vi "Lab Panel V4.83.vi"() -> ()   [LabVIEW 2013] (continued)
                        n911 = Number To Decimal String(number=w1505) -> (decimal integer string=w1518:string)  [unwired: 1 in]
                        n912 = Number To Decimal String(number=w1504) -> (decimal integer string=w1517:string)  [unwired: 1 in]
                        n913 = Number To Decimal String(number=w1503) -> (decimal integer string=w1516:string)  [unwired: 1 in]
                        n914 = Build Array(w1507, w1506, w1518, w1517, w1516) -> (w1515:string[])
                        n915 = TDMS Set Properties(5:w1515, 7:w1509, 11:w1519) -> ()  [unwired: 3 in, 4 out]
                      }
                      frame #3 {
                        w1521 = 0.0
                        n916 = local read "DISP LAB05-2"() -> (w1523:T4)
                        n917 = Bundle(cluster=w1523, "CYCLE"=w1521, "MINS"=w1521, "STATUS"="RUN") -> (w1522:T4)
                        n918 = local write "DISP LAB05-2"(w1522) -> ()
                      }
                      frame #4 {
                        n919 = local read "SIG LAB05-2"() -> (w1526:T2)
                        n920 = local read "TEMP START LAB05-2"() -> (w1528:cluster{"TL":dbl, "TN":dbl})
                        n921 = Unbundle(w1526) -> ("Tmp Live"=w1525:dbl, "Tmp Neut"=w1524:dbl)  [unwired: 3 out]
                        n922 = Bundle(cluster=w1528, "TL"=w1525, "TN"=w1524) -> (w1527:cluster{"TL":dbl, "TN":dbl})
                        n923 = local write "TEMP START LAB05-2"(w1527) -> ()
                      }
                    }
                  }
                }
              }
            }
            n924 = local write "data file error"(w580) -> ()
          }
          frame #4 {
            # "check if test cycles reached for cycle tests, if so then test pass"
            n925 = stacked-sequence {
              tunnel: w1548 -> [_ _ _ _ _ _ _ _ _ _]
              tunnel: w1547 -> [_ _ _ _ _ _ _ _ _ _]
              tunnel: w1546 -> [_ _ _ _ _ _ _ _ _ _]
              tunnel: w1545 -> [_ _ _ _ _ _ _ _ _ _]
              tunnel: w1544 -> [_ _ _ _ _ _ _ _ _ _]
              tunnel: w1543 -> [_ _ _ _ _ _ _ _ _ _]
              tunnel: w1542 -> [_ _ _ _ _ _ _ _ _ _]
              tunnel: w1541 -> [_ _ _ _ _ _ _ _ _ _]
              tunnel: w1540 -> [_ _ _ _ _ _ _ _ _ _]
              tunnel: w1539 -> [_ _ _ _ _ _ _ _ _ _]
              tunnel: w1538 -> [w1554 _ _ _ _ _ _ _ _ _]
              tunnel: w1537 -> [_ w1589 _ _ _ _ _ _ _ _]
              tunnel: w1536 -> [_ _ w1629 _ _ _ _ _ _ _]
              tunnel: w1535 -> [_ _ _ w1669 _ _ _ _ _ _]
              tunnel: w1534 -> [_ _ _ _ w1709 _ _ _ _ _]
              tunnel: w1533 -> [_ _ _ _ _ w1749 _ _ _ _]
              tunnel: w1532 -> [_ _ _ _ _ _ w1789 _ _ _]
              tunnel: w1531 -> [_ _ _ _ _ _ _ w1829 _ _]
              tunnel: w1530 -> [_ _ _ _ _ _ _ _ w1869 _]
              tunnel: w1529 -> [_ _ _ _ _ _ _ _ _ w1909]
              frame #0 {
                # "LAB01-1"
                n926 = Less?(x=w1554, y=2) -> (x < y?=w1552:bool)
                n927 = local read "DISP LAB01-1"() -> (w1555:T4)
                n928 = Unbundle(w1555) -> ("STATUS"=w1549:string)  [unwired: 2 out]
                n929 = Equal?(x=w1549, y="RUN") -> (x = y?=w1551:bool)
                n930 = And(x=w1551, y=w1552) -> (x .and. y?=w1550:bool)
                n931 = case shown="True" w1550 {
                  tunnel: w1555 -> [_ w1560]
                  tunnel: w1554 -> [_ w1564]
                  frame False {
                  }
                  frame True {
                    n932 = local read "SET LAB01-1"() -> (w1566:T5)
                    n933 = local read "TDMS LAB01-1"() -> (w1559:refnum<k34>)
                    n934 = Unbundle(w1566) -> ("CYCLES"=w1557:dbl, "T-RISE mins"=w1563:dbl)  [unwired: 3 out]
                    n935 = case shown="\"CYCLE TEST\"" w1564 {
                      tunnel: w1563 -> [_ _ w1573]
                      tunnel: [w1568 w1570 w1573] -> w1562
                      tunnel: w1557 -> [w1568 w1570 _]
                      tunnel: ["CHART PASS" "CYCLE PASS" "T-RISE PASS"] -> w1561
                      frame "CHART TEST", Default {
                      }
                      frame "CYCLE TEST" {
                      }
                      frame "T-RISE TEST" {
                      }
                    }
                    n936 = Unbundle(w1560) -> ("CYCLE"=w1565:dbl)  [unwired: 2 out]
                    n937 = Increment(x=w1557) -> (x+1=w1558:dbl)
                    n938 = Greater Or Equal?(x=w1565, y=w1558) -> (x >= y?=w1567:bool)
                    n939 = case shown="True" w1567 {
                      tunnel: w1562 -> [w1577 _]
                      tunnel: w1561 -> [w1576 _]
                      tunnel: w1560 -> [w1575 _]
                      tunnel: w1559 -> [w1574 _]
                      frame True {
                        n940 = stacked-sequence {
                          tunnel: w1577 -> [w1581 _]
                          tunnel: w1576 -> [w1579 w1585]
                          tunnel: w1575 -> [_ w1588]
                          tunnel: w1574 -> [w1578 _]
                          frame #0 {
                            n941 = Build Array(w1579) -> (w1582:string[])
                            n942 = Build Array(w1581) -> (w1580:dbl[])
                            n943 = TDMS Write(0:w1578, 5:"TEST PASS", 7:w1582, 9:w1580) -> (15:w1584:errorcluster)  [unwired: 2 in, 3 out]
                            n944 = local write "data file error"(w1584) -> ()
                          }
                          frame #1 {
                            n945 = Bundle(cluster=w1588, "STATUS"=w1585) -> (w1586:T4)  [unwired: 2 in]
                            n946 = local write "RESULT LAB01-1"(TRUE) -> ()
                            n947 = local write "DISP LAB01-1"(w1586) -> ()
                          }
                        }
                      }
                      frame False {
                      }
                    }
                  }
                }
              }
              frame #1 {
                # "LAB01-2"
                n948 = Less?(x=w1589, y=2) -> (x < y?=w1592:bool)
                n949 = local read "DISP LAB01-2"() -> (w1594:T4)
                n950 = Unbundle(w1594) -> ("STATUS"=w1595:string)  [unwired: 2 out]
                n951 = Equal?(x=w1595, y="RUN") -> (x = y?=w1591:bool)
                n952 = And(x=w1591, y=w1592) -> (x .and. y?=w1590:bool)
                n953 = case shown="True" w1590 {
                  tunnel: w1594 -> [_ w1600]
                  tunnel: w1589 -> [_ w1604]
                  frame False {
                  }
                  frame True {
                    n954 = local read "SET LAB01-2"() -> (w1606:T5)
                    n955 = local read "TDMS LAB01-2"() -> (w1599:refnum<k34>)
                    n956 = Unbundle(w1606) -> ("CYCLES"=w1597:dbl, "T-RISE mins"=w1603:dbl)  [unwired: 3 out]
                    n957 = case shown="\"T-RISE TEST\"" w1604 {
                      tunnel: w1603 -> [_ _ w1613]
                      tunnel: [w1608 w1610 w1613] -> w1602
                      tunnel: w1597 -> [w1608 w1610 _]
                      tunnel: ["CHART PASS" "CYCLE PASS" "T-RISE PASS"] -> w1601
                      frame "CHART TEST", Default {
                      }
                      frame "CYCLE TEST" {
                      }
                      frame "T-RISE TEST" {
                      }
                    }
                    n958 = Unbundle(w1600) -> ("CYCLE"=w1605:dbl)  [unwired: 2 out]
                    n959 = Increment(x=w1597) -> (x+1=w1598:dbl)
                    n960 = Greater Or Equal?(x=w1605, y=w1598) -> (x >= y?=w1607:bool)
                    n961 = case shown="True" w1607 {
                      tunnel: w1602 -> [w1617 _]
                      tunnel: w1601 -> [w1616 _]
                      tunnel: w1600 -> [w1615 _]
                      tunnel: w1599 -> [w1614 _]
                      frame True {
                        n962 = stacked-sequence {
                          tunnel: w1617 -> [w1621 _]
                          tunnel: w1616 -> [w1619 w1625]
                          tunnel: w1615 -> [_ w1628]
                          tunnel: w1614 -> [w1618 _]
                          frame #0 {
                            n963 = Build Array(w1619) -> (w1622:string[])
                            n964 = Build Array(w1621) -> (w1620:dbl[])
                            n965 = TDMS Write(0:w1618, 5:"TEST PASS", 7:w1622, 9:w1620) -> (15:w1624:errorcluster)  [unwired: 2 in, 3 out]
                            n966 = local write "data file error"(w1624) -> ()
                          }
                          frame #1 {
                            n967 = Bundle(cluster=w1628, "STATUS"=w1625) -> (w1626:T4)  [unwired: 2 in]
                            n968 = local write "RESULT LAB01-2"(TRUE) -> ()
                            n969 = local write "DISP LAB01-2"(w1626) -> ()
                          }
                        }
                      }
                      frame False {
                      }
                    }
                  }
                }
              }
              frame #2 {
                # "LAB02-1"
                n970 = Less?(x=w1629, y=2) -> (x < y?=w1632:bool)
                n971 = local read "DISP LAB02-1"() -> (w1634:T4)
                n972 = Unbundle(w1634) -> ("STATUS"=w1635:string)  [unwired: 2 out]
                n973 = Equal?(x=w1635, y="RUN") -> (x = y?=w1631:bool)
                n974 = And(x=w1631, y=w1632) -> (x .and. y?=w1630:bool)
                n975 = case shown="True" w1630 {
                  tunnel: w1634 -> [_ w1640]
                  tunnel: w1629 -> [_ w1644]
                  frame False {
                  }
                  frame True {
                    n976 = local read "SET LAB02-1"() -> (w1646:T5)
                    n977 = local read "TDMS LAB02-1"() -> (w1639:refnum<k34>)
                    n978 = Unbundle(w1640) -> ("CYCLE"=w1645:dbl)  [unwired: 2 out]
                    n979 = Unbundle(w1646) -> ("CYCLES"=w1637:dbl, "T-RISE mins"=w1643:dbl)  [unwired: 3 out]
                    n980 = case shown="\"T-RISE TEST\"" w1644 {
                      tunnel: w1643 -> [_ _ w1653]
                      tunnel: [w1648 w1650 w1653] -> w1642
                      tunnel: w1637 -> [w1648 w1650 _]
                      tunnel: ["CHART PASS" "CYCLE PASS" "T-RISE PASS"] -> w1641
                      frame "CHART TEST", Default {
                      }
                      frame "CYCLE TEST" {
                      }
                      frame "T-RISE TEST" {
                      }
                    }
                    n981 = Increment(x=w1637) -> (x+1=w1638:dbl)
                    n982 = Greater Or Equal?(x=w1645, y=w1638) -> (x >= y?=w1647:bool)
                    n983 = case shown="True" w1647 {
                      tunnel: w1642 -> [w1657 _]
                      tunnel: w1641 -> [w1656 _]
                      tunnel: w1640 -> [w1655 _]
                      tunnel: w1639 -> [w1654 _]
                      frame True {
                        n984 = stacked-sequence {
                          tunnel: w1657 -> [w1661 _]
                          tunnel: w1656 -> [w1659 w1665]
                          tunnel: w1655 -> [_ w1668]
                          tunnel: w1654 -> [w1658 _]
                          frame #0 {
                            n985 = Build Array(w1659) -> (w1662:string[])
                            n986 = Build Array(w1661) -> (w1660:dbl[])
                            n987 = TDMS Write(0:w1658, 5:"TEST PASS", 7:w1662, 9:w1660) -> (15:w1664:errorcluster)  [unwired: 2 in, 3 out]
                            n988 = local write "data file error"(w1664) -> ()
                          }
                          frame #1 {
                            n989 = Bundle(cluster=w1668, "STATUS"=w1665) -> (w1666:T4)  [unwired: 2 in]
                            n990 = local write "RESULT LAB02-1"(TRUE) -> ()
                            n991 = local write "DISP LAB02-1"(w1666) -> ()
                          }
                        }
                      }
                      frame False {
                      }
                    }
                  }
                }
              }
              frame #3 {
                # "LAB02-2"
                n992 = Less?(x=w1669, y=2) -> (x < y?=w1672:bool)
                n993 = local read "DISP LAB02-2"() -> (w1674:T4)
                n994 = Unbundle(w1674) -> ("STATUS"=w1675:string)  [unwired: 2 out]
                n995 = Equal?(x=w1675, y="RUN") -> (x = y?=w1671:bool)
                n996 = And(x=w1671, y=w1672) -> (x .and. y?=w1670:bool)
                n997 = case shown="True" w1670 {
                  tunnel: w1674 -> [_ w1680]
                  tunnel: w1669 -> [_ w1684]
                  frame False {
                  }
                  frame True {
                    n998 = local read "SET LAB02-2"() -> (w1686:T5)
                    n999 = local read "TDMS LAB02-2"() -> (w1679:refnum<k34>)
                    n1000 = Unbundle(w1680) -> ("CYCLE"=w1685:dbl)  [unwired: 2 out]
                    n1001 = Unbundle(w1686) -> ("CYCLES"=w1677:dbl, "T-RISE mins"=w1683:dbl)  [unwired: 3 out]
                    n1002 = case shown="\"T-RISE TEST\"" w1684 {
                      tunnel: w1683 -> [_ _ w1693]
                      tunnel: [w1688 w1690 w1693] -> w1682
                      tunnel: w1677 -> [w1688 w1690 _]
                      tunnel: ["CHART PASS" "CYCLE PASS" "T-RISE PASS"] -> w1681
                      frame "CHART TEST", Default {
                      }
                      frame "CYCLE TEST" {
                      }
                      frame "T-RISE TEST" {
                      }
                    }
                    n1003 = Increment(x=w1677) -> (x+1=w1678:dbl)
                    n1004 = Greater Or Equal?(x=w1685, y=w1678) -> (x >= y?=w1687:bool)
                    n1005 = case shown="True" w1687 {
                      tunnel: w1682 -> [w1697 _]
                      tunnel: w1681 -> [w1696 _]
                      tunnel: w1680 -> [w1695 _]
                      tunnel: w1679 -> [w1694 _]
                      frame True {
                        n1006 = stacked-sequence {
                          tunnel: w1697 -> [w1701 _]
                          tunnel: w1696 -> [w1699 w1705]
                          tunnel: w1695 -> [_ w1708]
                          tunnel: w1694 -> [w1698 _]
                          frame #0 {
                            n1007 = Build Array(w1699) -> (w1702:string[])
                            n1008 = Build Array(w1701) -> (w1700:dbl[])
                            n1009 = TDMS Write(0:w1698, 5:"TEST PASS", 7:w1702, 9:w1700) -> (15:w1704:errorcluster)  [unwired: 2 in, 3 out]
                            n1010 = local write "data file error"(w1704) -> ()
                          }
                          frame #1 {
                            n1011 = Bundle(cluster=w1708, "STATUS"=w1705) -> (w1706:T4)  [unwired: 2 in]
                            n1012 = local write "RESULT LAB02-2"(TRUE) -> ()
                            n1013 = local write "DISP LAB02-2"(w1706) -> ()
                          }
                        }
                      }
                      frame False {
                      }
                    }
                  }
                }
              }
              frame #4 {
                # "LAB03-1"
                n1014 = Less?(x=w1709, y=2) -> (x < y?=w1712:bool)
                n1015 = local read "DISP LAB03-1"() -> (w1714:T4)
                n1016 = Unbundle(w1714) -> ("STATUS"=w1715:string)  [unwired: 2 out]
                n1017 = Equal?(x=w1715, y="RUN") -> (x = y?=w1711:bool)
                n1018 = And(x=w1711, y=w1712) -> (x .and. y?=w1710:bool)
                n1019 = case shown="True" w1710 {
                  tunnel: w1714 -> [_ w1720]
                  tunnel: w1709 -> [_ w1724]
                  frame False {
                  }
                  frame True {
                    n1020 = local read "SET LAB03-1"() -> (w1726:T5)
                    n1021 = local read "TDMS LAB03-1"() -> (w1719:refnum<k34>)
                    n1022 = Unbundle(w1720) -> ("CYCLE"=w1725:dbl)  [unwired: 2 out]
                    n1023 = Unbundle(w1726) -> ("CYCLES"=w1717:dbl, "T-RISE mins"=w1723:dbl)  [unwired: 3 out]
                    n1024 = case shown="\"T-RISE TEST\"" w1724 {
                      tunnel: w1723 -> [_ _ w1733]
                      tunnel: [w1728 w1730 w1733] -> w1722
                      tunnel: w1717 -> [w1728 w1730 _]
                      tunnel: ["CHART PASS" "CYCLE PASS" "T-RISE PASS"] -> w1721
                      frame "CHART TEST", Default {
                      }
                      frame "CYCLE TEST" {
                      }
                      frame "T-RISE TEST" {
                      }
                    }
                    n1025 = Increment(x=w1717) -> (x+1=w1718:dbl)
                    n1026 = Greater Or Equal?(x=w1725, y=w1718) -> (x >= y?=w1727:bool)
                    n1027 = case shown="True" w1727 {
                      tunnel: w1722 -> [w1737 _]
                      tunnel: w1721 -> [w1736 _]
                      tunnel: w1720 -> [w1735 _]
                      tunnel: w1719 -> [w1734 _]
                      frame True {
                        n1028 = stacked-sequence {
                          tunnel: w1737 -> [w1741 _]
                          tunnel: w1736 -> [w1739 w1745]
                          tunnel: w1735 -> [_ w1748]
                          tunnel: w1734 -> [w1738 _]
                          frame #0 {
                            n1029 = Build Array(w1739) -> (w1742:string[])
                            n1030 = Build Array(w1741) -> (w1740:dbl[])
                            n1031 = TDMS Write(0:w1738, 5:"TEST PASS", 7:w1742, 9:w1740) -> (15:w1744:errorcluster)  [unwired: 2 in, 3 out]
                            n1032 = local write "data file error"(w1744) -> ()
                          }
                          frame #1 {
                            n1033 = Bundle(cluster=w1748, "STATUS"=w1745) -> (w1746:T4)  [unwired: 2 in]
                            n1034 = local write "RESULT LAB03-1"(TRUE) -> ()
                            n1035 = local write "DISP LAB03-1"(w1746) -> ()
                          }
                        }
                      }
                      frame False {
                      }
                    }
                  }
                }
              }
              frame #5 {
                # "LAB03-2"
                n1036 = Less?(x=w1749, y=2) -> (x < y?=w1752:bool)
                n1037 = local read "DISP LAB03-2"() -> (w1754:T4)
                n1038 = Unbundle(w1754) -> ("STATUS"=w1755:string)  [unwired: 2 out]
                n1039 = Equal?(x=w1755, y="RUN") -> (x = y?=w1751:bool)
                n1040 = And(x=w1751, y=w1752) -> (x .and. y?=w1750:bool)
                n1041 = case shown="True" w1750 {
                  tunnel: w1754 -> [_ w1760]
                  tunnel: w1749 -> [_ w1764]
                  frame False {
                  }
                  frame True {
                    n1042 = local read "SET LAB03-2"() -> (w1766:T5)
                    n1043 = local read "TDMS LAB03-2"() -> (w1759:refnum<k34>)
                    n1044 = Unbundle(w1760) -> ("CYCLE"=w1765:dbl)  [unwired: 2 out]
                    n1045 = Unbundle(w1766) -> ("CYCLES"=w1757:dbl, "T-RISE mins"=w1763:dbl)  [unwired: 3 out]
                    n1046 = case shown="\"T-RISE TEST\"" w1764 {
                      tunnel: w1763 -> [_ _ w1773]
                      tunnel: [w1768 w1770 w1773] -> w1762
                      tunnel: w1757 -> [w1768 w1770 _]
                      tunnel: ["CHART PASS" "CYCLE PASS" "T-RISE PASS"] -> w1761
                      frame "CHART TEST", Default {
                      }
                      frame "CYCLE TEST" {
                      }
                      frame "T-RISE TEST" {
                      }
                    }
                    n1047 = Increment(x=w1757) -> (x+1=w1758:dbl)
                    n1048 = Greater Or Equal?(x=w1765, y=w1758) -> (x >= y?=w1767:bool)
                    n1049 = case shown="True" w1767 {
                      tunnel: w1762 -> [w1777 _]
                      tunnel: w1761 -> [w1776 _]
                      tunnel: w1760 -> [w1775 _]
                      tunnel: w1759 -> [w1774 _]
                      frame True {
                        n1050 = stacked-sequence {
                          tunnel: w1777 -> [w1781 _]
                          tunnel: w1776 -> [w1779 w1785]
                          tunnel: w1775 -> [_ w1788]
                          tunnel: w1774 -> [w1778 _]
                          frame #0 {
                            n1051 = Build Array(w1779) -> (w1782:string[])
                            n1052 = Build Array(w1781) -> (w1780:dbl[])
                            n1053 = TDMS Write(0:w1778, 5:"TEST PASS", 7:w1782, 9:w1780) -> (15:w1784:errorcluster)  [unwired: 2 in, 3 out]
                            n1054 = local write "data file error"(w1784) -> ()
                          }
                          frame #1 {
                            n1055 = Bundle(cluster=w1788, "STATUS"=w1785) -> (w1786:T4)  [unwired: 2 in]
                            n1056 = local write "RESULT LAB03-2"(TRUE) -> ()
                            n1057 = local write "DISP LAB03-2"(w1786) -> ()
                          }
                        }
                      }
                      frame False {
                      }
                    }
                  }
                }
              }
              frame #6 {
                # "LAB04-1"
                n1058 = Less?(x=w1789, y=2) -> (x < y?=w1792:bool)
                n1059 = local read "DISP LAB04-1"() -> (w1794:T4)
                n1060 = Unbundle(w1794) -> ("STATUS"=w1795:string)  [unwired: 2 out]
                n1061 = Equal?(x=w1795, y="RUN") -> (x = y?=w1791:bool)
                n1062 = And(x=w1791, y=w1792) -> (x .and. y?=w1790:bool)
                n1063 = case shown="True" w1790 {
                  tunnel: w1794 -> [_ w1800]
                  tunnel: w1789 -> [_ w1804]
                  frame False {
                  }
                  frame True {
                    n1064 = local read "SET LAB04-1"() -> (w1806:T5)
                    n1065 = local read "TDMS LAB04-1"() -> (w1799:refnum<k34>)
                    n1066 = Unbundle(w1800) -> ("CYCLE"=w1805:dbl)  [unwired: 2 out]
                    n1067 = Unbundle(w1806) -> ("CYCLES"=w1797:dbl, "T-RISE mins"=w1803:dbl)  [unwired: 3 out]
                    n1068 = case shown="\"T-RISE TEST\"" w1804 {
                      tunnel: w1803 -> [_ _ w1813]
                      tunnel: [w1808 w1810 w1813] -> w1802
                      tunnel: w1797 -> [w1808 w1810 _]
                      tunnel: ["CHART PASS" "CYCLE PASS" "T-RISE PASS"] -> w1801
                      frame "CHART TEST", Default {
                      }
                      frame "CYCLE TEST" {
                      }
                      frame "T-RISE TEST" {
                      }
                    }
                    n1069 = Increment(x=w1797) -> (x+1=w1798:dbl)
                    n1070 = Greater Or Equal?(x=w1805, y=w1798) -> (x >= y?=w1807:bool)
                    n1071 = case shown="True" w1807 {
                      tunnel: w1802 -> [w1817 _]
                      tunnel: w1801 -> [w1816 _]
                      tunnel: w1800 -> [w1815 _]
                      tunnel: w1799 -> [w1814 _]
                      frame True {
                        n1072 = stacked-sequence {
                          tunnel: w1817 -> [w1821 _]
                          tunnel: w1816 -> [w1819 w1825]
                          tunnel: w1815 -> [_ w1828]
                          tunnel: w1814 -> [w1818 _]
                          frame #0 {
                            n1073 = Build Array(w1819) -> (w1822:string[])
                            n1074 = Build Array(w1821) -> (w1820:dbl[])
                            n1075 = TDMS Write(0:w1818, 5:"TEST PASS", 7:w1822, 9:w1820) -> (15:w1824:errorcluster)  [unwired: 2 in, 3 out]
                            n1076 = local write "data file error"(w1824) -> ()
                          }
                          frame #1 {
                            n1077 = Bundle(cluster=w1828, "STATUS"=w1825) -> (w1826:T4)  [unwired: 2 in]
                            n1078 = local write "RESULT LAB04-1"(TRUE) -> ()
                            n1079 = local write "DISP LAB04-1"(w1826) -> ()
                          }
                        }
                      }
                      frame False {
                      }
                    }
                  }
                }
              }
              frame #7 {
                # "LAB04-2"
                n1080 = Less?(x=w1829, y=2) -> (x < y?=w1832:bool)
                n1081 = local read "DISP LAB04-2"() -> (w1834:T4)
                n1082 = Unbundle(w1834) -> ("STATUS"=w1835:string)  [unwired: 2 out]
                n1083 = Equal?(x=w1835, y="RUN") -> (x = y?=w1831:bool)
                n1084 = And(x=w1831, y=w1832) -> (x .and. y?=w1830:bool)
                n1085 = case shown="True" w1830 {
                  tunnel: w1834 -> [_ w1840]
                  tunnel: w1829 -> [_ w1844]
                  frame False {
                  }
                  frame True {
                    n1086 = local read "SET LAB04-2"() -> (w1846:T5)
                    n1087 = local read "TDMS LAB04-2"() -> (w1839:refnum<k34>)
                    n1088 = Unbundle(w1840) -> ("CYCLE"=w1845:dbl)  [unwired: 2 out]
                    n1089 = Unbundle(w1846) -> ("CYCLES"=w1837:dbl, "T-RISE mins"=w1843:dbl)  [unwired: 3 out]
                    n1090 = case shown="\"T-RISE TEST\"" w1844 {
                      tunnel: w1843 -> [_ _ w1853]
                      tunnel: [w1848 w1850 w1853] -> w1842
                      tunnel: w1837 -> [w1848 w1850 _]
                      tunnel: ["CHART PASS" "CYCLE PASS" "T-RISE PASS"] -> w1841
                      frame "CHART TEST", Default {
                      }
                      frame "CYCLE TEST" {
                      }
                      frame "T-RISE TEST" {
                      }
                    }
                    n1091 = Increment(x=w1837) -> (x+1=w1838:dbl)
                    n1092 = Greater Or Equal?(x=w1845, y=w1838) -> (x >= y?=w1847:bool)
                    n1093 = case shown="True" w1847 {
                      tunnel: w1842 -> [w1857 _]
                      tunnel: w1841 -> [w1856 _]
                      tunnel: w1840 -> [w1855 _]
                      tunnel: w1839 -> [w1854 _]
                      frame True {
                        n1094 = stacked-sequence {
                          tunnel: w1857 -> [w1861 _]
                          tunnel: w1856 -> [w1859 w1865]
                          tunnel: w1855 -> [_ w1868]
                          tunnel: w1854 -> [w1858 _]
                          frame #0 {
                            n1095 = Build Array(w1859) -> (w1862:string[])
                            n1096 = Build Array(w1861) -> (w1860:dbl[])
                            n1097 = TDMS Write(0:w1858, 5:"TEST PASS", 7:w1862, 9:w1860) -> (15:w1864:errorcluster)  [unwired: 2 in, 3 out]
                            n1098 = local write "data file error"(w1864) -> ()
                          }
                          frame #1 {
                            n1099 = Bundle(cluster=w1868, "STATUS"=w1865) -> (w1866:T4)  [unwired: 2 in]
                            n1100 = local write "RESULT LAB04-2"(TRUE) -> ()
                            n1101 = local write "DISP LAB04-2"(w1866) -> ()
                          }
                        }
                      }
                      frame False {
                      }
                    }
                  }
                }
              }
              frame #8 {
                # "LAB05-1"
                n1102 = Less?(x=w1869, y=2) -> (x < y?=w1872:bool)
                n1103 = local read "DISP LAB05-1"() -> (w1874:T4)
                n1104 = Unbundle(w1874) -> ("STATUS"=w1875:string)  [unwired: 2 out]
                n1105 = Equal?(x=w1875, y="RUN") -> (x = y?=w1871:bool)
                n1106 = And(x=w1871, y=w1872) -> (x .and. y?=w1870:bool)
                n1107 = case shown="True" w1870 {
                  tunnel: w1874 -> [_ w1880]
                  tunnel: w1869 -> [_ w1884]
                  frame False {
                  }
                  frame True {
                    n1108 = local read "SET LAB05-1"() -> (w1886:T5)
                    n1109 = local read "TDMS LAB05-1"() -> (w1879:refnum<k34>)
                    n1110 = Unbundle(w1880) -> ("CYCLE"=w1885:dbl)  [unwired: 2 out]
                    n1111 = Unbundle(w1886) -> ("CYCLES"=w1877:dbl, "T-RISE mins"=w1883:dbl)  [unwired: 3 out]
                    n1112 = case shown="\"T-RISE TEST\"" w1884 {
                      tunnel: w1883 -> [_ _ w1893]
                      tunnel: [w1888 w1890 w1893] -> w1882
                      tunnel: w1877 -> [w1888 w1890 _]
                      tunnel: ["CHART PASS" "CYCLE PASS" "T-RISE PASS"] -> w1881
                      frame "CHART TEST", Default {
                      }
                      frame "CYCLE TEST" {
                      }
                      frame "T-RISE TEST" {
                      }
                    }
                    n1113 = Increment(x=w1877) -> (x+1=w1878:dbl)
                    n1114 = Greater Or Equal?(x=w1885, y=w1878) -> (x >= y?=w1887:bool)
                    n1115 = case shown="True" w1887 {
                      tunnel: w1882 -> [w1897 _]
                      tunnel: w1881 -> [w1896 _]
                      tunnel: w1880 -> [w1895 _]
                      tunnel: w1879 -> [w1894 _]
                      frame True {
                        n1116 = stacked-sequence {
                          tunnel: w1897 -> [w1901 _]
                          tunnel: w1896 -> [w1899 w1905]
                          tunnel: w1895 -> [_ w1908]
                          tunnel: w1894 -> [w1898 _]
                          frame #0 {
                            n1117 = Build Array(w1899) -> (w1902:string[])
                            n1118 = Build Array(w1901) -> (w1900:dbl[])
                            n1119 = TDMS Write(0:w1898, 5:"TEST PASS", 7:w1902, 9:w1900) -> (15:w1904:errorcluster)  [unwired: 2 in, 3 out]
                            n1120 = local write "data file error"(w1904) -> ()
                          }
                          frame #1 {
                            n1121 = Bundle(cluster=w1908, "STATUS"=w1905) -> (w1906:T4)  [unwired: 2 in]
                            n1122 = local write "RESULT LAB05-1"(TRUE) -> ()
                            n1123 = local write "DISP LAB05-1"(w1906) -> ()
                          }
                        }
                      }
                      frame False {
                      }
                    }
                  }
                }
              }
              frame #9 {
                # "LAB05-2"
                n1124 = Less?(x=w1909, y=2) -> (x < y?=w1912:bool)
                n1125 = local read "DISP LAB05-2"() -> (w1914:T4)
                n1126 = Unbundle(w1914) -> ("STATUS"=w1915:string)  [unwired: 2 out]
                n1127 = Equal?(x=w1915, y="RUN") -> (x = y?=w1911:bool)
                n1128 = And(x=w1911, y=w1912) -> (x .and. y?=w1910:bool)
                n1129 = case shown="True" w1910 {
                  tunnel: w1914 -> [_ w1920]
                  tunnel: w1909 -> [_ w1924]
                  frame False {
                  }
                  frame True {
                    n1130 = local read "SET LAB05-2"() -> (w1926:T5)
                    n1131 = local read "TDMS LAB05-2"() -> (w1919:refnum<k34>)
                    n1132 = Unbundle(w1920) -> ("CYCLE"=w1925:dbl)  [unwired: 2 out]
                    n1133 = Unbundle(w1926) -> ("CYCLES"=w1917:dbl, "T-RISE mins"=w1923:dbl)  [unwired: 3 out]
                    n1134 = case shown="\"T-RISE TEST\"" w1924 {
                      tunnel: w1923 -> [_ _ w1933]
                      tunnel: [w1928 w1930 w1933] -> w1922
                      tunnel: w1917 -> [w1928 w1930 _]
                      tunnel: ["CHART PASS" "CYCLE PASS" "T-RISE PASS"] -> w1921
                      frame "CHART TEST", Default {
                      }
                      frame "CYCLE TEST" {
                      }
                      frame "T-RISE TEST" {
                      }
                    }
                    n1135 = Increment(x=w1917) -> (x+1=w1918:dbl)
                    n1136 = Greater Or Equal?(x=w1925, y=w1918) -> (x >= y?=w1927:bool)
                    n1137 = case shown="True" w1927 {
                      tunnel: w1922 -> [w1937 _]
                      tunnel: w1921 -> [w1936 _]
                      tunnel: w1920 -> [w1935 _]
                      tunnel: w1919 -> [w1934 _]
                      frame True {
                        n1138 = stacked-sequence {
                          tunnel: w1937 -> [w1941 _]
                          tunnel: w1936 -> [w1939 w1945]
                          tunnel: w1935 -> [_ w1948]
                          tunnel: w1934 -> [w1938 _]
                          frame #0 {
                            n1139 = Build Array(w1939) -> (w1942:string[])
                            n1140 = Build Array(w1941) -> (w1940:dbl[])
                            n1141 = TDMS Write(0:w1938, 5:"TEST PASS", 7:w1942, 9:w1940) -> (15:w1944:errorcluster)  [unwired: 2 in, 3 out]
                            n1142 = local write "data file error"(w1944) -> ()
                          }
                          frame #1 {
                            n1143 = Bundle(cluster=w1948, "STATUS"=w1945) -> (w1946:T4)  [unwired: 2 in]
                            n1144 = local write "RESULT LAB05-2"(TRUE) -> ()
                            n1145 = local write "DISP LAB05-2"(w1946) -> ()
                          }
                        }
                      }
                      frame False {
                      }
                    }
                  }
                }
              }
            }
          }
          frame #5 {
            # "check if test cycles reached for temperature rise test"
            n1146 = stacked-sequence {
              tunnel: w1978 -> [_ _ _ _ _ _ _ _ _ _]
              tunnel: w1977 -> [_ _ _ _ _ _ _ _ _ _]
              tunnel: w1976 -> [_ _ _ _ _ _ _ _ _ _]
              tunnel: w1975 -> [_ _ _ _ _ _ _ _ _ _]
              tunnel: w1974 -> [_ _ _ _ _ _ _ _ _ _]
              tunnel: w1973 -> [_ _ _ _ _ _ _ _ _ _]
              tunnel: w1972 -> [_ _ _ _ _ _ _ _ _ _]
              tunnel: w1971 -> [_ _ _ _ _ _ _ _ _ _]
              tunnel: w1970 -> [_ _ _ _ _ _ _ _ _ _]
              tunnel: w1969 -> [_ _ _ _ _ _ _ _ _ _]
              tunnel: w1968 -> [w1984 _ _ _ _ _ _ _ _ _]
              tunnel: w1958 -> [w1979 _ _ _ _ _ _ _ _ _]
              tunnel: w1967 -> [_ w2010 _ _ _ _ _ _ _ _]
              tunnel: w1966 -> [_ _ w2040 _ _ _ _ _ _ _]
              tunnel: w1965 -> [_ _ _ w2070 _ _ _ _ _ _]
              tunnel: w1964 -> [_ _ _ _ w2100 _ _ _ _ _]
              tunnel: w1963 -> [_ _ _ _ _ w2130 _ _ _ _]
              tunnel: w1962 -> [_ _ _ _ _ _ w2160 _ _ _]
              tunnel: w1961 -> [_ _ _ _ _ _ _ w2190 _ _]
              tunnel: w1960 -> [_ _ _ _ _ _ _ _ w2220 _]
              tunnel: w1959 -> [_ _ _ _ _ _ _ _ _ w2250]
              tunnel: w1957 -> [_ w2009 _ _ _ _ _ _ _ _]
              tunnel: w1956 -> [_ _ w2039 _ _ _ _ _ _ _]
              tunnel: w1955 -> [_ _ _ w2069 _ _ _ _ _ _]
              tunnel: w1954 -> [_ _ _ _ w2099 _ _ _ _ _]
              tunnel: w1953 -> [_ _ _ _ _ w2129 _ _ _ _]
              tunnel: w1952 -> [_ _ _ _ _ _ w2159 _ _ _]
              tunnel: w1951 -> [_ _ _ _ _ _ _ w2189 _ _]
              tunnel: w1950 -> [_ _ _ _ _ _ _ _ w2219 _]
              tunnel: w1949 -> [_ _ _ _ _ _ _ _ _ w2249]
              frame #0 {
                # "LAB01-1"
                n1147 = Equal?(x=w1984, y=2) -> (x = y?=w1982:bool)
                n1148 = local read "DISP LAB01-1"() -> (w1985:T4)
                n1149 = Unbundle(w1985) -> ("STATUS"=w1986:string)  [unwired: 2 out]
                n1150 = Equal?(x=w1986, y="RUN") -> (x = y?=w1981:bool)
                n1151 = And(x=w1981, y=w1982) -> (x .and. y?=w1980:bool)
                n1152 = case shown="True" w1980 {
                  tunnel: w1985 -> [_ w1989]
                  tunnel: w1979 -> [_ w1992]
                  frame False {
                  }
                  frame True {
                    n1153 = local read "SET LAB01-1"() -> (w1991:T5)
                    n1154 = local read "TDMS LAB01-1"() -> (w1988:refnum<k34>)
                    n1155 = Unbundle(w1989) -> ("CYCLE"=w1993:dbl)  [unwired: 2 out]
                    n1156 = Unbundle(w1991) -> ("T-RISE mins"=w1990:dbl)  [unwired: 4 out]
                    n1157 = Greater Or Equal?(x=w1993, y=w1992) -> (x >= y?=w1994:bool)
                    n1158 = case shown="True" w1994 {
                      tunnel: w1990 -> [w1997 _]
                      tunnel: w1989 -> [w1996 _]
                      tunnel: w1988 -> [w1995 _]
                      frame True {
                        n1159 = stacked-sequence {
                          tunnel: w1997 -> [w2000 _]
                          tunnel: w1996 -> [_ w2005]
                          tunnel: w1995 -> [w1998 _]
                          frame #0 {
                            n1160 = Build Array("T-RISE") -> (w2002:string[])
                            n1161 = Build Array(w2000) -> (w2001:dbl[])
                            n1162 = TDMS Write(0:w1998, 5:"TEST PASS", 7:w2002, 9:w2001) -> (15:w2004:errorcluster)  [unwired: 2 in, 3 out]
                            n1163 = local write "data file error"(w2004) -> ()
                          }
                          frame #1 {
                            n1164 = Bundle(cluster=w2005, "STATUS"="T-RISE PASS") -> (w2007:T4)  [unwired: 2 in]
                            n1165 = local write "RESULT LAB01-1"(TRUE) -> ()
                            n1166 = local write "DISP LAB01-1"(w2007) -> ()
                          }
                        }
                      }
                      frame False {
                      }
                    }
                  }
                }
              }
              frame #1 {
                # "LAB01-2"
                n1167 = Equal?(x=w2010, y=2) -> (x = y?=w2013:bool)
                n1168 = local read "DISP LAB01-2"() -> (w2015:T4)
                n1169 = Unbundle(w2015) -> ("STATUS"=w2016:string)  [unwired: 2 out]
                n1170 = Equal?(x=w2016, y="RUN") -> (x = y?=w2012:bool)
                n1171 = And(x=w2012, y=w2013) -> (x .and. y?=w2011:bool)
                n1172 = case shown="True" w2011 {
                  tunnel: w2015 -> [_ w2019]
                  tunnel: w2009 -> [_ w2022]
                  frame False {
                  }
                  frame True {
                    n1173 = local read "SET LAB01-2"() -> (w2021:T5)
                    n1174 = local read "TDMS LAB01-2"() -> (w2018:refnum<k34>)
                    n1175 = Unbundle(w2019) -> ("CYCLE"=w2023:dbl)  [unwired: 2 out]
                    n1176 = Unbundle(w2021) -> ("T-RISE mins"=w2020:dbl)  [unwired: 4 out]
                    n1177 = Greater Or Equal?(x=w2023, y=w2022) -> (x >= y?=w2024:bool)
                    n1178 = case shown="True" w2024 {
                      tunnel: w2020 -> [w2027 _]
                      tunnel: w2019 -> [w2026 _]
                      tunnel: w2018 -> [w2025 _]
                      frame True {
                        n1179 = stacked-sequence {
                          tunnel: w2027 -> [w2030 _]
                          tunnel: w2026 -> [_ w2035]
                          tunnel: w2025 -> [w2028 _]
                          frame #0 {
                            n1180 = Build Array("T-RISE") -> (w2032:string[])
                            n1181 = Build Array(w2030) -> (w2031:dbl[])
                            n1182 = TDMS Write(0:w2028, 5:"TEST PASS", 7:w2032, 9:w2031) -> (15:w2034:errorcluster)  [unwired: 2 in, 3 out]
                            n1183 = local write "data file error"(w2034) -> ()
                          }
                          frame #1 {
                            n1184 = Bundle(cluster=w2035, "STATUS"="T-RISE PASS") -> (w2037:T4)  [unwired: 2 in]
                            n1185 = local write "RESULT LAB01-2"(TRUE) -> ()
                            n1186 = local write "DISP LAB01-2"(w2037) -> ()
                          }
                        }
                      }
                      frame False {
                      }
                    }
                  }
                }
              }
              frame #2 {
                # "LAB02-1"
                n1187 = Equal?(x=w2040, y=2) -> (x = y?=w2043:bool)
                n1188 = local read "DISP LAB02-1"() -> (w2045:T4)
                n1189 = Unbundle(w2045) -> ("STATUS"=w2046:string)  [unwired: 2 out]
                n1190 = Equal?(x=w2046, y="RUN") -> (x = y?=w2042:bool)
                n1191 = And(x=w2042, y=w2043) -> (x .and. y?=w2041:bool)
                n1192 = case shown="True" w2041 {
                  tunnel: w2045 -> [_ w2049]
                  tunnel: w2039 -> [_ w2052]
                  frame False {
                  }
                  frame True {
                    n1193 = local read "SET LAB02-1"() -> (w2051:T5)
                    n1194 = local read "TDMS LAB02-1"() -> (w2048:refnum<k34>)
                    n1195 = Unbundle(w2049) -> ("CYCLE"=w2053:dbl)  [unwired: 2 out]
                    n1196 = Unbundle(w2051) -> ("T-RISE mins"=w2050:dbl)  [unwired: 4 out]
                    n1197 = Greater Or Equal?(x=w2053, y=w2052) -> (x >= y?=w2054:bool)
                    n1198 = case shown="True" w2054 {
                      tunnel: w2050 -> [w2057 _]
                      tunnel: w2049 -> [w2056 _]
                      tunnel: w2048 -> [w2055 _]
                      frame True {
                        n1199 = stacked-sequence {
                          tunnel: w2057 -> [w2060 _]
                          tunnel: w2056 -> [_ w2065]
                          tunnel: w2055 -> [w2058 _]
                          frame #0 {
                            n1200 = Build Array("T-RISE") -> (w2062:string[])
                            n1201 = Build Array(w2060) -> (w2061:dbl[])
                            n1202 = TDMS Write(0:w2058, 5:"TEST PASS", 7:w2062, 9:w2061) -> (15:w2064:errorcluster)  [unwired: 2 in, 3 out]
                            n1203 = local write "data file error"(w2064) -> ()
                          }
                          frame #1 {
                            n1204 = Bundle(cluster=w2065, "STATUS"="T-RISE PASS") -> (w2067:T4)  [unwired: 2 in]
                            n1205 = local write "RESULT LAB02-1"(TRUE) -> ()
                            n1206 = local write "DISP LAB02-1"(w2067) -> ()
                          }
                        }
                      }
                      frame False {
                      }
                    }
                  }
                }
              }
              frame #3 {
                # "LAB02-2"
                n1207 = Equal?(x=w2070, y=2) -> (x = y?=w2073:bool)
                n1208 = local read "DISP LAB02-2"() -> (w2075:T4)
                n1209 = Unbundle(w2075) -> ("STATUS"=w2076:string)  [unwired: 2 out]
                n1210 = Equal?(x=w2076, y="RUN") -> (x = y?=w2072:bool)
                n1211 = And(x=w2072, y=w2073) -> (x .and. y?=w2071:bool)
                n1212 = case shown="True" w2071 {
                  tunnel: w2075 -> [_ w2079]
                  tunnel: w2069 -> [_ w2082]
                  frame False {
                  }
                  frame True {
                    n1213 = local read "SET LAB02-2"() -> (w2081:T5)
                    n1214 = local read "TDMS LAB02-2"() -> (w2078:refnum<k34>)
                    n1215 = Unbundle(w2079) -> ("CYCLE"=w2083:dbl)  [unwired: 2 out]
                    n1216 = Unbundle(w2081) -> ("T-RISE mins"=w2080:dbl)  [unwired: 4 out]
                    n1217 = Greater Or Equal?(x=w2083, y=w2082) -> (x >= y?=w2084:bool)
                    n1218 = case shown="True" w2084 {
                      tunnel: w2080 -> [w2087 _]
                      tunnel: w2079 -> [w2086 _]
                      tunnel: w2078 -> [w2085 _]
                      frame True {
                        n1219 = stacked-sequence {
                          tunnel: w2087 -> [w2090 _]
                          tunnel: w2086 -> [_ w2095]
                          tunnel: w2085 -> [w2088 _]
                          frame #0 {
                            n1220 = Build Array("T-RISE") -> (w2092:string[])
                            n1221 = Build Array(w2090) -> (w2091:dbl[])
                            n1222 = TDMS Write(0:w2088, 5:"TEST PASS", 7:w2092, 9:w2091) -> (15:w2094:errorcluster)  [unwired: 2 in, 3 out]
                            n1223 = local write "data file error"(w2094) -> ()
                          }
                          frame #1 {
                            n1224 = Bundle(cluster=w2095, "STATUS"="T-RISE PASS") -> (w2097:T4)  [unwired: 2 in]
                            n1225 = local write "RESULT LAB02-2"(TRUE) -> ()
                            n1226 = local write "DISP LAB02-2"(w2097) -> ()
                          }
                        }
                      }
                      frame False {
                      }
                    }
                  }
                }
              }
              frame #4 {
                # "LAB03-1"
                n1227 = Equal?(x=w2100, y=2) -> (x = y?=w2103:bool)
                n1228 = local read "DISP LAB03-1"() -> (w2105:T4)
                n1229 = Unbundle(w2105) -> ("STATUS"=w2106:string)  [unwired: 2 out]
                n1230 = Equal?(x=w2106, y="RUN") -> (x = y?=w2102:bool)
                n1231 = And(x=w2102, y=w2103) -> (x .and. y?=w2101:bool)
                n1232 = case shown="True" w2101 {
                  tunnel: w2105 -> [_ w2109]
                  tunnel: w2099 -> [_ w2112]
                  frame False {
                  }
                  frame True {
                    n1233 = local read "SET LAB03-1"() -> (w2111:T5)
                    n1234 = local read "TDMS LAB03-1"() -> (w2108:refnum<k34>)
                    n1235 = Unbundle(w2109) -> ("CYCLE"=w2113:dbl)  [unwired: 2 out]
                    n1236 = Unbundle(w2111) -> ("T-RISE mins"=w2110:dbl)  [unwired: 4 out]
                    n1237 = Greater Or Equal?(x=w2113, y=w2112) -> (x >= y?=w2114:bool)
                    n1238 = case shown="True" w2114 {
                      tunnel: w2110 -> [w2117 _]
                      tunnel: w2109 -> [w2116 _]
                      tunnel: w2108 -> [w2115 _]
                      frame True {
                        n1239 = stacked-sequence {
                          tunnel: w2117 -> [w2120 _]
                          tunnel: w2116 -> [_ w2125]
                          tunnel: w2115 -> [w2118 _]
                          frame #0 {
                            n1240 = Build Array("T-RISE") -> (w2122:string[])
                            n1241 = Build Array(w2120) -> (w2121:dbl[])
                            n1242 = TDMS Write(0:w2118, 5:"TEST PASS", 7:w2122, 9:w2121) -> (15:w2124:errorcluster)  [unwired: 2 in, 3 out]
                            n1243 = local write "data file error"(w2124) -> ()
                          }
                          frame #1 {
                            n1244 = Bundle(cluster=w2125, "STATUS"="T-RISE PASS") -> (w2127:T4)  [unwired: 2 in]
                            n1245 = local write "RESULT LAB03-1"(TRUE) -> ()
                            n1246 = local write "DISP LAB03-1"(w2127) -> ()
                          }
                        }
                      }
                      frame False {
                      }
                    }
                  }
                }
              }
              frame #5 {
                # "LAB03-2"
